vi "CreateLVAddonJSONfile.vi"() -> ()   [LabVIEW 2021]
uses:
  <vilib>/Wiresmith Technology/G CLI/CLI Class/CLI.lvclass
panel:
  in  "Arguments":string[](array[string])
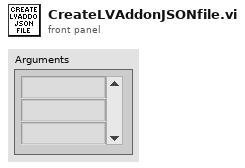
[diagram p1: front panel]
types:
  T1 = enum32{"Invalid", "Standard", "Closed", "Hidden", "Minimized", "Maximized"}
  T2 = enum16{"open", "replace", "create", "open or create", "replace or create", "replace or create with confirmation"}
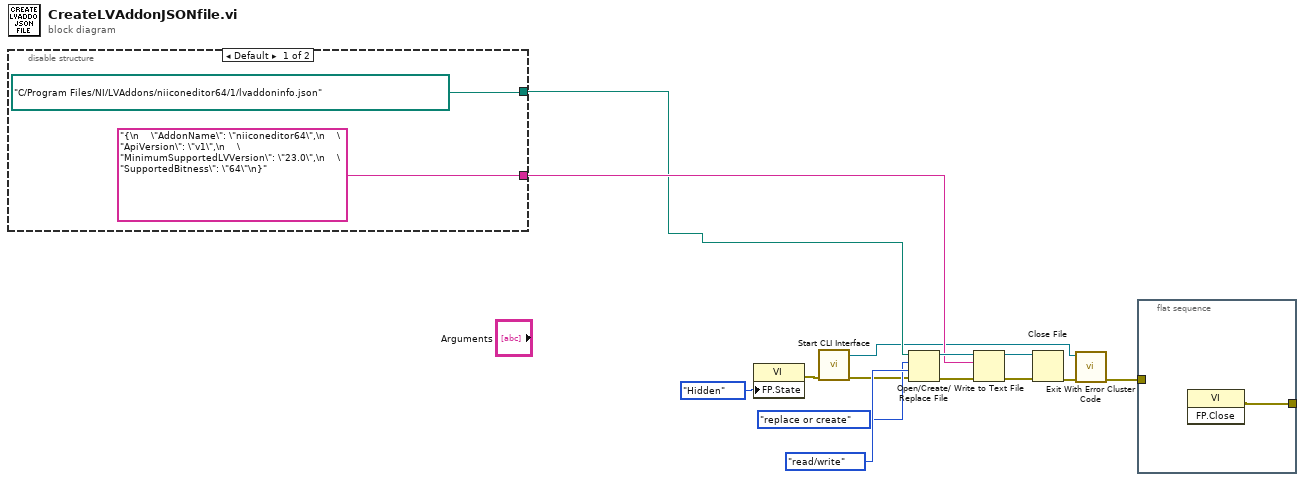
[diagram p0: block diagram]
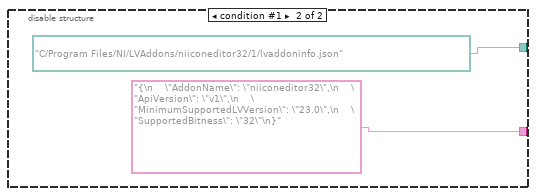
[diagram p2: hidden frame]
diagram:
  n1 = disable-structure shown="Default" {
    disable-tunnel: [path "C:/Program Files/NI/LVAddons/niiconeditor64/1/lvaddoninfo.json" ("Destination[i] Paths (Absolute)") path "C:/Program Files/NI/LVAddons/niiconeditor32/1/lvaddoninfo.json" ("Destination[i] Paths (Absolute)")] -> w7
    disable-tunnel: ["{\n    \"AddonName\": \"niiconeditor64\",\n    \"ApiVersion\": \"v1\",\n    \"MinimumSupportedLVVersion\": \"23.0\",\n    \"SupportedBitness\": \"64\"\n}" ("Tag Name") "{\n    \"AddonName\": \"niiconeditor32\",\n    \"ApiVersion\": \"v1\",\n    \"MinimumSupportedLVVersion\": \"23.0\",\n    \"SupportedBitness\": \"32\"\n}" ("Tag Name")] -> w8
    frame condition #0 (active) {
    }
    frame condition #1 {
    }
  }
  n2 = property class="VI"("FP.State"=T1."Hidden" ("Front Panel Window:State")) -> (error out=w5:errorcluster)  [unwired: 2 in, 1 out]
  n3 = call <vilib>:"Start CLI Interface.vi"("error in (no error)"=w5) -> ("error out"=w4:errorcluster, "CLI out"=w2:refnum<class "CLI.lvclass">)  [unwired: 7 in, 2 out]
  n4 = Open/Create/Replace File(file path (use dialog)=w7, error in=w4, operation (0:open)=T2."replace or create", access (0:read/write)=enum16{"read/write", "read-only", "write-only"}."read/write") -> (refnum out=w13:refnum<file>, error out=w10:errorcluster)  [unwired: 2 in, 1 out]
  n5 = Write to Text File(file (use dialog)=w13, text=w8, error in=w10) -> (refnum out=w14:refnum<file>, error out=w9:errorcluster)  [unwired: 1 in, 1 out]
  n6 = Close File(refnum=w14, error in=w9) -> (error out=w3:errorcluster)  [unwired: 1 out]
  n7 = call <vilib>:"Exit With Error Cluster Code.vi"("error in (no error)"=w3, "CLI in"=w2) -> ("error out"=w1:errorcluster)  [unwired: 9 in]
  n8 = flat-sequence {
    tunnel: [w19] -> _
    tunnel: w1 -> [_]
    frame #0 {
      n9 = invoke class="VI" method="FP.Close"() -> (error out=w19:errorcluster)  [unwired: 3 in, 2 out]
    }
  }
